vi "System_Main.vi"() -> ()   [LabVIEW 2019]
uses:
  Subsys01/Subsys01_Global.vi
  Subsys02/Subsys02_Global.vi
panel:
  in  "control_lock":bool caption="Control"
  in  "stop_all":bool caption="open_THCD_400"
  in  "start_all":bool caption="open_THCD_400"
  in  "open_S02":bool caption="open_THCD_400"
  in  "open_S01":bool caption="open_THCD_400"
  out "S02_V02":dbl
  out "S02_V01":dbl
  out "S02_ST":u32(colorbox)
  out "S01_ST":u32(colorbox)
  in  "stop":bool
  out "S01_V01":i64
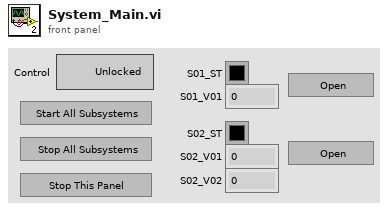
[diagram p1: front panel]
types:
  T1 = enum8{"Enabled", "Disabled", "Disabled and Grayed Out"}
  T2 = enum32{"Bad", "Idle", "Run top level", "Running"}
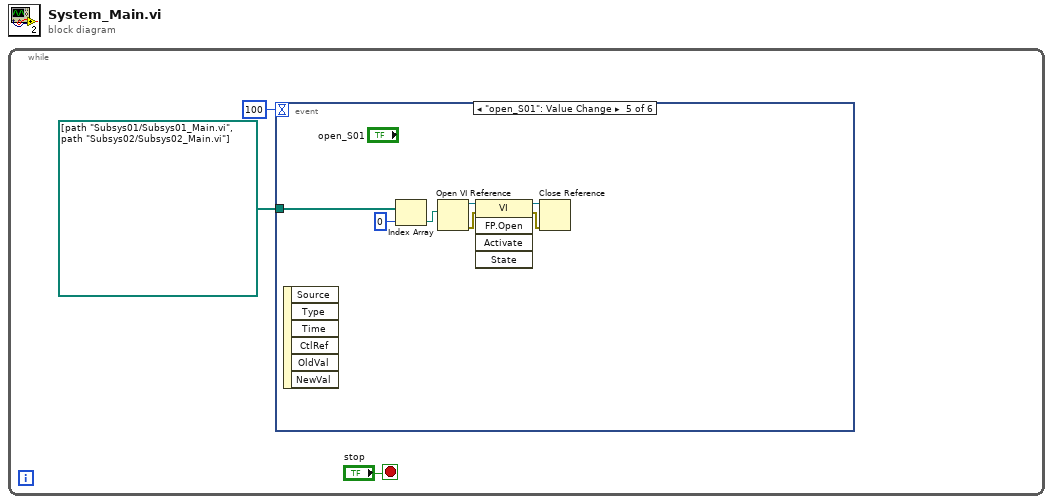
[diagram p0: block diagram]
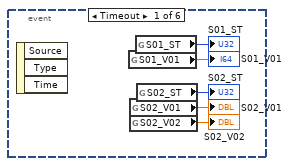
[diagram p2: hidden frame]
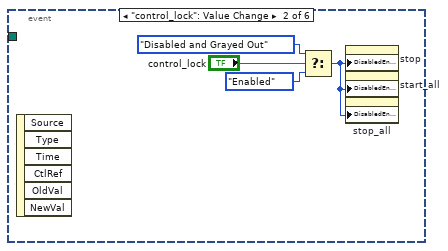
[diagram p3: hidden frame]
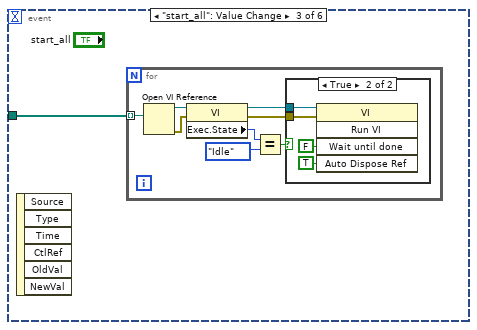
[diagram p4: hidden frame]
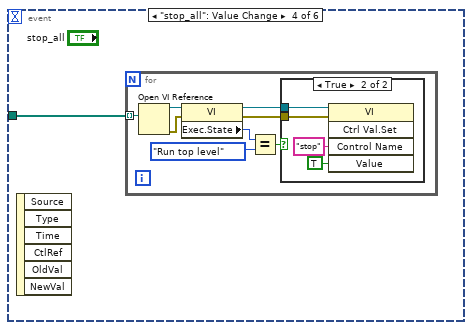
[diagram p6: hidden frame]
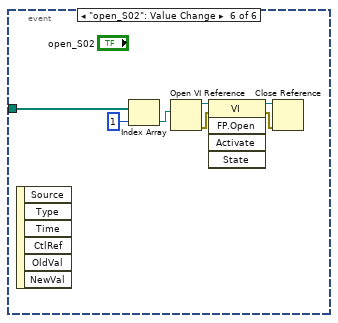
[diagram p8: hidden frame]
diagram:
  n1 = while {
    stop <- "stop" stop-if-true
    n2 = event shown="[4] \"open_S01\": Value Change" {
      selector: _ -> [_ _ _ _ _ _]
      dyn-events: _ -> [_ _ _ _ _ _]
      timeout: 100 -> [_ _ _ _ _ _]
      tunnel: path[] [path "Subsys01/Subsys01_Main.vi", path "Subsys02/Subsys02_Main.vi"] -> [_ _ w13 w26 w41 w47]
      event Timeout {
        n3 = event-data() -> ()  [unwired: 1 in, 3 out]
        n4 = global read "Subsys01_Global.vi" "S01_V01"() -> (→"S01_V01":dbl)
        n5 = global read "Subsys02_Global.vi" "S02_V01"() -> (→"S02_V01":dbl)
        n6 = global read "Subsys02_Global.vi" "S02_V02"() -> (→"S02_V02":dbl)
        n7 = global read "Subsys01_Global.vi" "S01_ST"() -> (→"S01_ST":u32)
        n8 = global read "Subsys02_Global.vi" "S02_ST"() -> (→"S02_ST":u32)
      }
      event "control_lock": Value Change {
        n9 = event-data() -> ()  [unwired: 1 in, 6 out]
        n10 = Select(t=T1."Disabled and Grayed Out" ("Disabled"), s="control_lock", f=T1."Enabled" ("Disabled")) -> (s? t:f=w9:T1)
        n11 = property on="stop" class="Bool"("DisabledEnum"=w9) -> ()  [unwired: 2 in, 2 out]
        n12 = property on="start_all" class="Bool"("DisabledEnum"=w9) -> ()  [unwired: 2 in, 2 out]
        n13 = property on="stop_all" class="Bool"("DisabledEnum"=w9) -> ()  [unwired: 2 in, 2 out]
      }
      event "start_all": Value Change {
        n14 = event-data() -> ()  [unwired: 1 in, 6 out]
        n15 = for {
          tunnel: w13 -> [w14] mode=indexing
          n16 = Open VI Reference(vi path=w14) -> (vi reference=w21:refnum<vi>, error out=w20:errorcluster)  [unwired: 5 in]
          n17 = property class="VI"(reference=w21, error in=w20) -> (reference out=w19:refnum<vi>, error out=w18:errorcluster, "Exec.State"=w17:T2)
          n18 = Equal?(x=w17, y=T2."Idle" ("Execution:State")) -> (x = y?=w15:bool)
          n19 = case shown="True" w15 {
            tunnel: w19 -> [_ w23]
            tunnel: w18 -> [_ w22]
            frame False {
            }
            frame True {
              n20 = invoke class="VI" method="Run VI"(reference=w23, error in=w22, "Wait until done"=FALSE ("Wait Until Done"), "Auto Dispose Ref"=TRUE ("Auto Dispose Reference")) -> ()  [unwired: 1 in, 5 out]
            }
          }
        }
      }
      event "stop_all": Value Change {
        n21 = event-data() -> ()  [unwired: 1 in, 6 out]
        n22 = for {
          tunnel: w26 -> [w27] mode=indexing
          n23 = Open VI Reference(vi path=w27) -> (vi reference=w34:refnum<vi>, error out=w33:errorcluster)  [unwired: 5 in]
          n24 = property class="VI"(reference=w34, error in=w33) -> (reference out=w32:refnum<vi>, error out=w31:errorcluster, "Exec.State"=w30:T2)
          n25 = Equal?(x=w30, y=T2."Run top level" ("Execution:State")) -> (x = y?=w28:bool)
          n26 = case shown="True" w28 {
            tunnel: w32 -> [_ w37]
            tunnel: w31 -> [_ w36]
            frame False {
            }
            frame True {
              n27 = invoke class="VI" method="Ctrl Val.Set"(reference=w37, error in=w36, "Control Name"="stop", "Value"=TRUE ("Auto Dispose Reference")) -> ()  [unwired: 1 in, 5 out]
            }
          }
        }
      }
      event "open_S01": Value Change {
        n28 = event-data() -> ()  [unwired: 1 in, 6 out]
        n29 = Index Array(array=w41, index=0) -> (element=w39:path)
        n30 = Open VI Reference(vi path=w39) -> (vi reference=w43:refnum<vi>, error out=w44:errorcluster)  [unwired: 5 in]
        n31 = invoke class="VI" method="FP.Open"(reference=w43, error in=w44) -> (reference out=w42:refnum<vi>, error out=w45:errorcluster)  [unwired: 3 in, 3 out]
        n32 = Close Reference(reference=w42, error in (no error)=w45) -> ()  [unwired: 1 out]
      }
      event "open_S02": Value Change {
        n33 = event-data() -> ()  [unwired: 1 in, 6 out]
        n34 = Index Array(array=w47, index=1) -> (element=w46:path)
        n35 = Open VI Reference(vi path=w46) -> (vi reference=w50:refnum<vi>, error out=w51:errorcluster)  [unwired: 5 in]
        n36 = invoke class="VI" method="FP.Open"(reference=w50, error in=w51) -> (reference out=w49:refnum<vi>, error out=w52:errorcluster)  [unwired: 3 in, 3 out]
        n37 = Close Reference(reference=w49, error in (no error)=w52) -> ()  [unwired: 1 out]
      }
    }
  }
